vi "Example.vi"() -> ()   [LabVIEW 2020]
panel:
  out "CT":i32
  out "Q":bool
  in  "CTD":bool
  in  "CTU":bool
  in  "PV":i32
  in  "Reset":bool
  in  "Reset":bool
  in  "PV":i32
  in  "CTD":bool
  out "CT":i32
  out "Q":bool
  in  "Reset":bool
  out "Q":bool
  out "CT":i32
  in  "PV":i32
  in  "CTU":bool
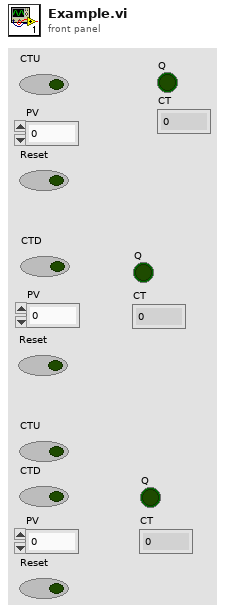
[diagram p1: front panel]
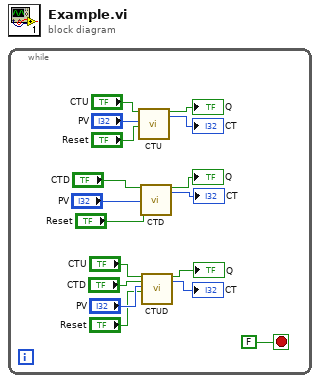
[diagram p0: block diagram]
diagram:
  n1 = while {
    stop <- FALSE stop-if-true
    n2 = call "CTU.vi"("CTU"="CTU", "PV"="PV", "Reset"="Reset") -> ("Q"=→"Q":bool, "CT"=→"CT":i32)  [unwired: 15 in]
    n3 = call "CTD.vi"("CTD"="CTD", "PV"="PV", "Reset"="Reset") -> ("Q"=→"Q":bool, "CT"=→"CT":i32)  [unwired: 15 in]
    n4 = call "CTUD.vi"("CTU"="CTU", "CTD"="CTD", "PV"="PV", "Reset"="Reset") -> ("Q"=→"Q":bool, "CT"=→"CT":i32)  [unwired: 14 in]
  }
